vi "ClassPanel.vi"(8 "error in (no error)":errorcluster caption="entrée d'erreur (pas d'erreur)", 11 "CoboltMLD.lvclass":refnum<class "CoboltMLD.lvclass">) -> (0 "error out":errorcluster caption="sortie d'erreur", 3 "CoboltMLD.lvclass Out":refnum<class "CoboltMLD.lvclass">)   [LabVIEW 2019, in "CoboltMLD.lvclass"]
uses:
  CoboltMLD.lvclass
  CoboltModes.ctl
  C:/Programmes Labview/LabscanV1A/DevicesClass/BaseDevice/BaseDevice.lvclass
  <userlib>/TaikoLaser/PDLM_TaggedValueList.ctl
  <userlib>/TaikoLaser/PDLM_TaggedValue.ctl
  <userlib>/TaikoLaser/PDLM_Tag.ctl
  BaseDevice/BaseDevice.lvclass/BaseDevice.ctl
  BaseDevice/ClassQueueMess.ctl
  BaseDevice/Accessor/GetBaseDataPath.vi
  BaseDevice/Accessor/GetClassEvent.vi
panel:
  out "MaxSetpoint":dbl
  in  "Paused":bool
  out "Hours":dbl
  in  "AMod":bool
  out "Fault":string
  in  "DMod":bool
  out "Act Current":dbl caption="Current (mA)" min=0.1 step=0.1 format="%#.3f"
  out "ForceDis":bool caption="Force disconnect"
  out "Error":bool
  out "JournalPath":path
  in  "Con/Disc.":bool
  out "Interlock":bool
  out "Temp":dbl caption="Temp (C)" min=0.1 step=0.1 format="%#.1f"
  out "Act Power":dbl caption="Power (mW)" min=0.1 step=0.1 format="%#.3f"
  in  "Update":bool
  in  "Mode":T1 caption="Laser Mode"
  in  "LaserOn":bool caption="Laser On"
  out "KeyLock":bool
  in  "Setp_Pc":dbl=1.0 caption="Setpoint(%)" min=0.0 max=100.0 step=0.01 format="%#.1f"
  in  "MainProgQ":refnum<queue>
  in  "MainProgQEvent":refnum<user-event>
  in  "Acq":bool
  in  "Stop":bool
  in  "Setp_Un":dbl=200.0 caption="Setpoint(mW)" min=0.0 max=200.0 step=0.01 format="%#.1f"
  out "Init Program":bool
  # "Cobolt Laser"
  # "this MUST labeled with class name"
  # "this MUST be present and labeled \"Stop\" and \"Acq\""
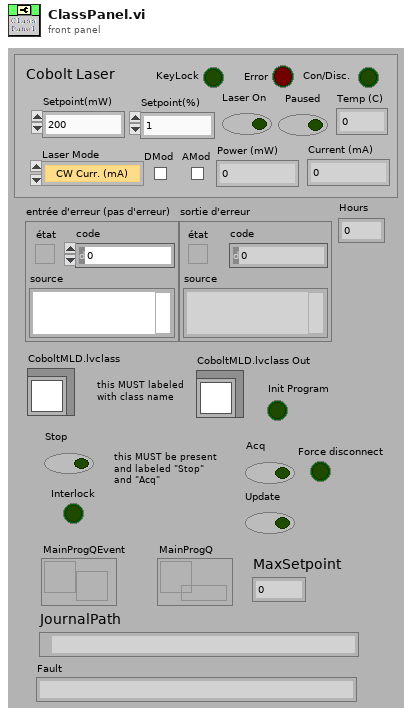
[diagram p1: front panel]
types:
  T1 = typedef "CoboltModes.ctl" = enum16{"CW Curr. (mA)", "CW Pow. (mW)", "Curr. Mod. (mA)", "Pow. Mod. (mW)"}
  T2 = typedef "PDLM_Tag.ctl" = u32
  T3 = typedef "PDLM_TaggedValueList.ctl" = T4[]
  T4 = typedef "PDLM_TaggedValue.ctl" = cluster{"Tag":T2, "Value":u32}
  T5 = typedef "ClassQueueMess.ctl" = u16
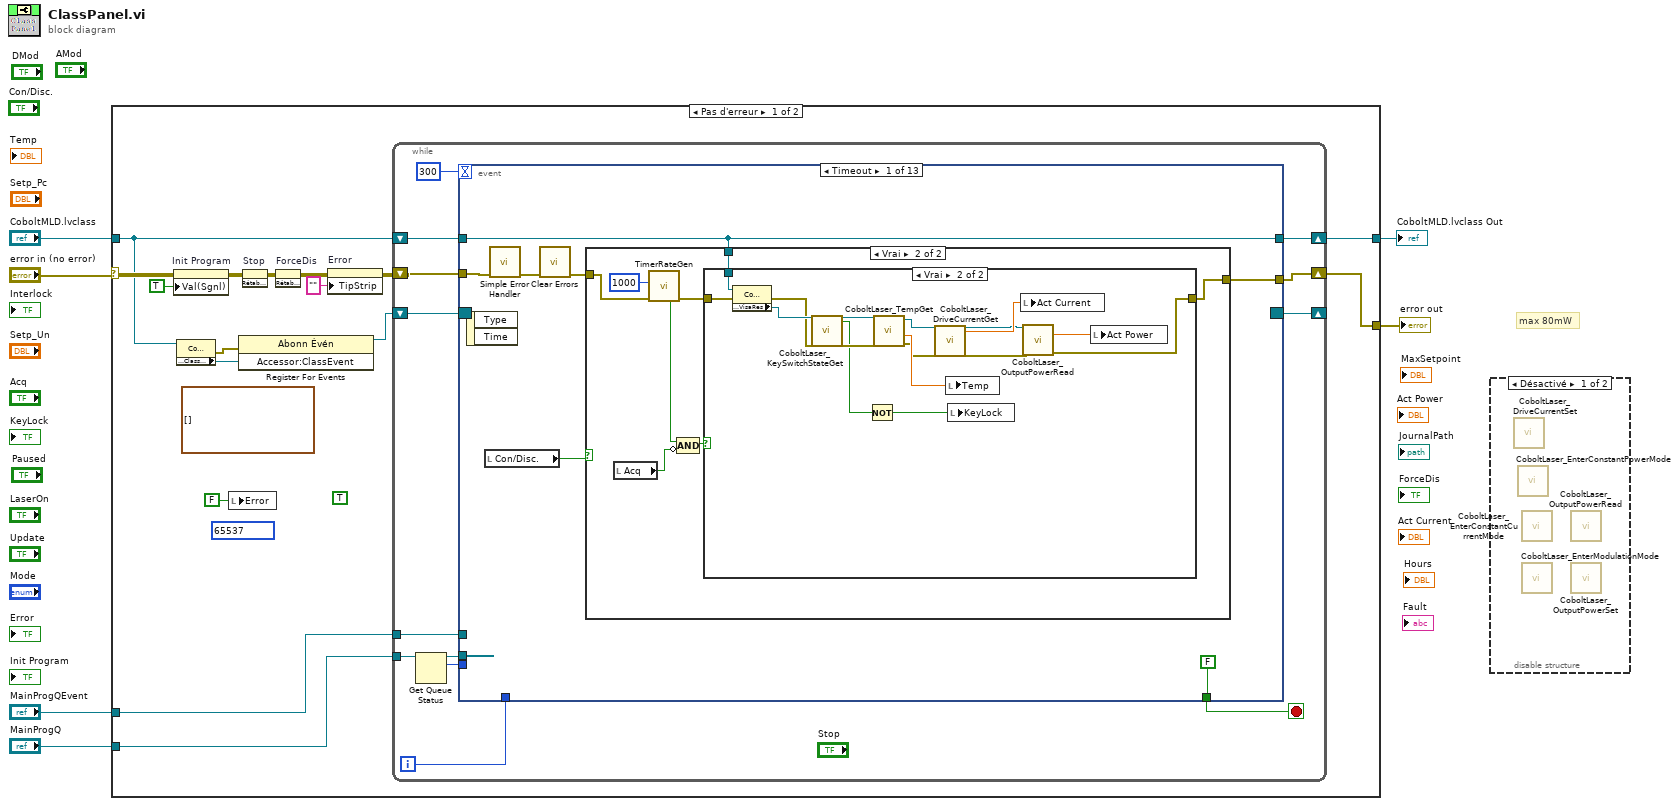
[diagram p0: block diagram]
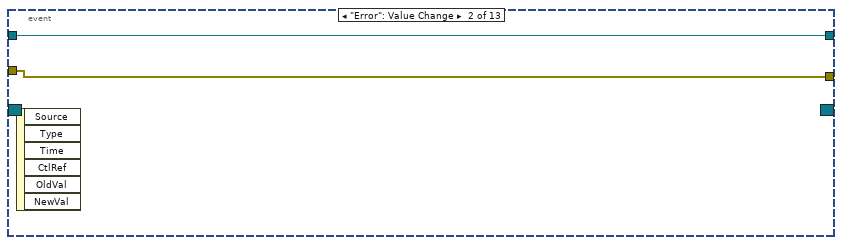
[diagram p5: hidden frame]
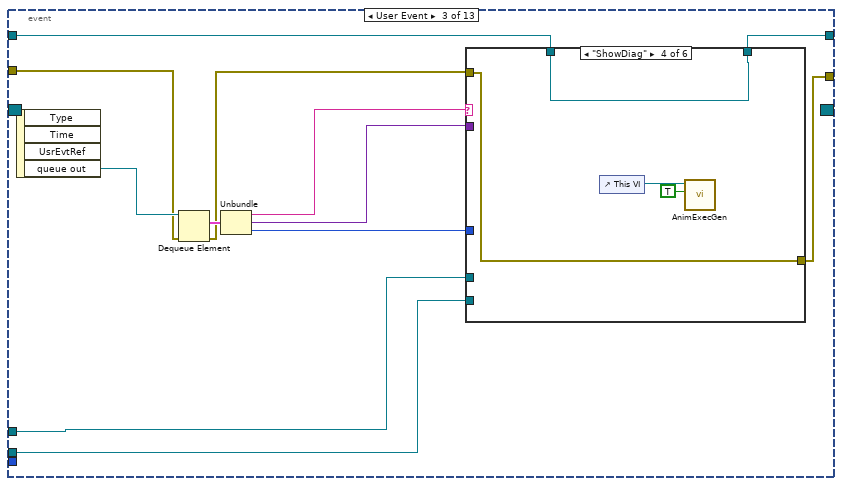
[diagram p6: hidden frame]
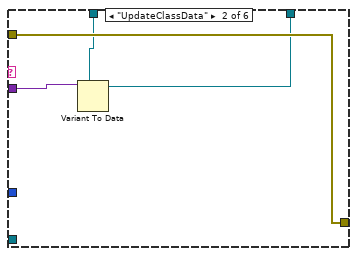
[diagram p8: hidden frame]
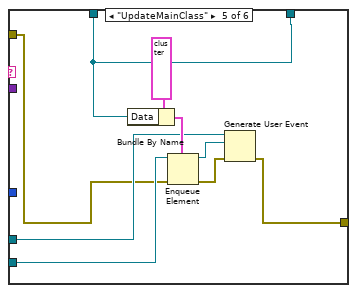
[diagram p10: hidden frame]
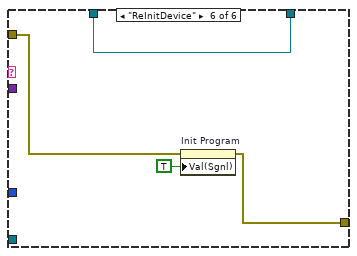
[diagram p11: hidden frame]
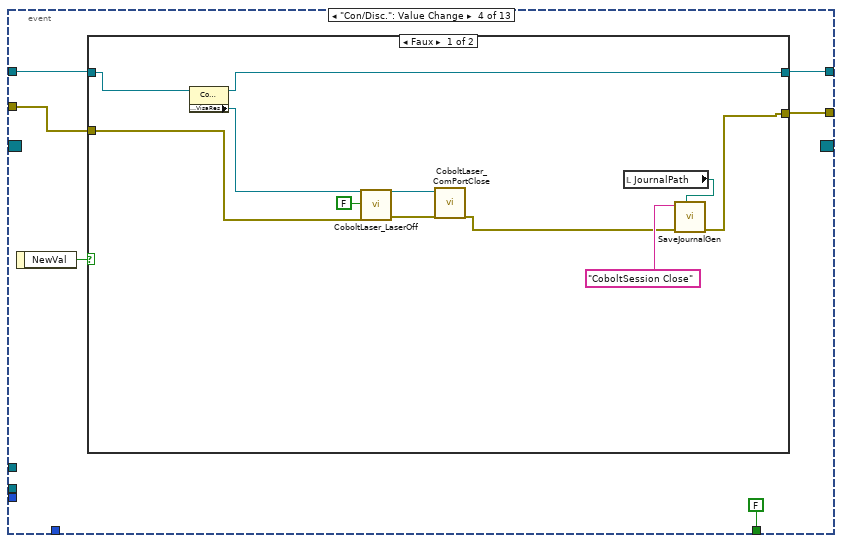
[diagram p12: hidden frame]
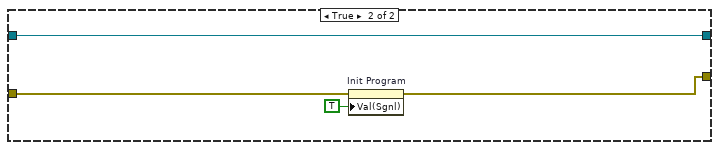
[diagram p13: hidden frame]
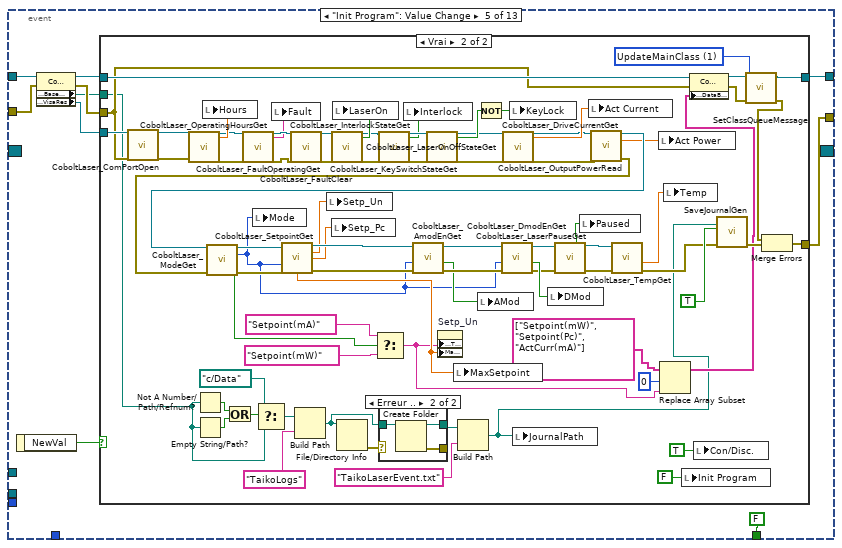
[diagram p14: hidden frame]
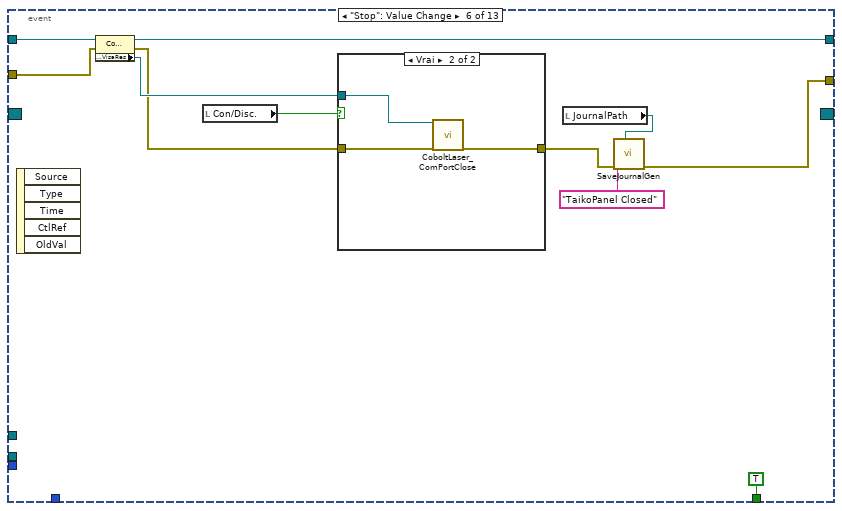
[diagram p17: hidden frame]
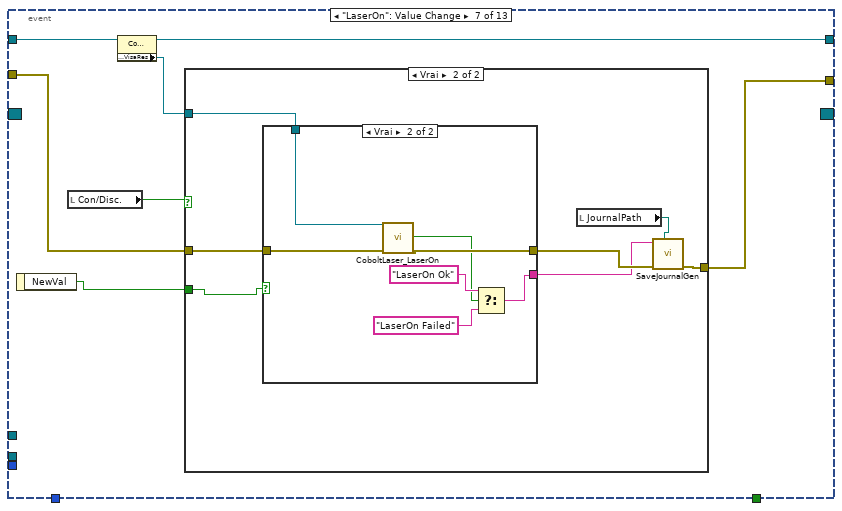
[diagram p19: hidden frame]
diagram:
  # "max 80mW"
  n1 = case shown="Pas d'erreur" "error in (no error)" {
    selector: "error in (no error)" -> [w11 w381]
    tunnel: [w22 w381] -> w5
    tunnel: "CoboltMLD.lvclass" -> [w16 w380]
    tunnel: [w20 w380] -> w3
    tunnel: "MainProgQEvent" -> [w14 _]
    tunnel: "MainProgQ" -> [w13 _]
    frame No Error {
      (unwired) TRUE ("ForceDis")
      (unwired) T2 65537 items=["NONE"=0, "Locked"=16, "SoftLock"=17, "KeyLock"=18, "Class_IV_Lock"=20, "Interlock"=24, "LaserMode"=32, "LDH_PulsePowerTable"=33, "TriggerMode"=48, "TriggerLevelRaw"=64, "TriggerLevelRawLoLimit"=65, "TriggerLevelRawHiLimit"=66, "TriggerLevel"=72, "TriggerLevelLoLimit"=73, "TriggerLevelHiLimit"=74, "FastGate"=80, "FastGateImp"=96, "SlowGate"=112, "TargetTempRaw"=144, "TargetTempRawLoLimit"=145, "TargetTempRawHiLimit"=146, "CurrentTempRaw"=148, "CaseTempRaw"=149, "TargetTemp"=152, "TargetTempLoLimit"=153, "TargetTempHiLimit"=154, "CurrentTemp"=156, "CaseTemp"=157, "TempScale"=159, "Frequency"=168, "FrequencyLoLimit"=169, "FrequencyHiLimit"=170, "PulsePowerRaw"=176, "PulsePowerRawLoLimit"=177, "PulsePowerRawHiLimit"=178, "PulsePowerPermille"=180, "PulseShape"=181, "PulsePower"=184, "PulsePowerLoLimit"=185, "PulsePowerHiLimit"=186, "PulsePowerNanowatt"=188, "PulsePowerVoltage"=190, "PulseEnergy"=191, "CwPowerRaw"=192, "CwPowerRawLoLimit"=193, "CwPowerRawHiLimit"=194, "CwPowerPermille"=196, "CwPower"=200, "CwPowerLoLimit"=201, "CwPowerHiLimit"=202, "CwPowerMicroWatt"=204, "BurstLen"=208, "BurstPeriod"=224, "LDH_Fan"=240, "UI_Exclusive"=256] ("Tag")
      (unwired) T3 [] ("TaggedValueList")
      n2 = property on="Init Program" class="Bool (strict)"(error in=w11, "Val(Sgnl)"=TRUE ("Valeur (Signalisation)")) -> (error out=w19:errorcluster)  [unwired: 1 in, 1 out]
      n3 = property class="CoboltMLD.lvclass"(reference=w16) -> (error out=w18:errorcluster, "Accessor:ClassEvent"=w17:refnum<user-event>)  [unwired: 1 in, 1 out]
      n4 = local write "Error"(FALSE ("Error")) -> ()
      n5 = register-events(error in=w18, w17) -> (reference out=w15:refnum<event-registration>)  [unwired: 1 in, 1 out]
      n6 = invoke on="Stop" class="Bool (strict)" method="RétablirValParDéfaut"(error in=w19) -> (error out=w10:errorcluster)  [unwired: 2 in, 2 out]
      n7 = invoke on="ForceDis" class="Bool (strict)" method="RétablirValParDéfaut"(error in=w10) -> (error out=w9:errorcluster)  [unwired: 2 in, 2 out]
      n8 = property on="Error" class="Bool (strict)"(error in=w9, "TipStrip"="" ("Info-bulle")) -> (error out=w8:errorcluster)  [unwired: 1 in, 1 out]
      n9 = while {
        shift-right: [w33] -> w22
        shift-left: w8 -> [w34]
        shift-right: [w32] -> w20
        shift-left: w16 -> [w26]
        shift-right: [w30] -> _
        shift-left: w15 -> [w31]
        tunnel: w14 -> [w29]
        tunnel: w13 -> [w28]
        i -> [w27]
        stop <- w25 stop-if-true
        n10 = Get Queue Status(queue=w28) -> (queue out=w24:refnum<queue>, # pending remove=w23:i32)  [unwired: 2 in, 6 out]
        n11 = event shown="[0] Timeout" {
          selector: w31 -> [_ _ _ _ _ _ _ _ _ _ _ _ _]
          dyn-events: [_ _ _ _ _ _ _ _ _ _ _ _ _] -> w30
          timeout: 300 -> [_ _ _ _ _ _ _ _ _ _ _ _ _]
          tunnel: w34 -> [w40 w69 w72 w112 w132 w224 w244 w269 w300 w312 w325 w335 w349]
          tunnel: [w37 w69 w76 w109 w137 w229 w242 w271 w298 w310 w323 w334 w346] -> w33
          tunnel: w26 -> [w36 w70 w82 w110 w135 w232 w243 w272 w299 w311 w324 w337 w350]
          tunnel: [FALSE _ _ FALSE FALSE TRUE _ _ _ _ _ _ _] -> w25
          tunnel: [w36 w70 w75 w108 w134 w226 w241 w270 w299 w311 w324 w337 w343] -> w32
          tunnel: w29 -> [_ _ w74 _ _ _ _ _ _ _ _ _ _]
          tunnel: w24 -> [_ _ w73 _ _ _ _ _ _ _ _ _ _]
          tunnel: w27 -> [_ _ _ _ _ _ _ _ _ _ _ _ _]
          tunnel: w23 -> [_ _ _ _ _ _ _ _ _ _ _ _ _]
          event Timeout {
            n12 = event-data() -> ()  [unwired: 1 in, 2 out]
            n13 = local read "Con/Disc."() -> (w38:bool)
            n14 = call <vilib>:"Simple Error Handler.vi"("error in (no error)"=w40) -> ("error out"=w41:errorcluster)  [unwired: 4 in, 4 out]
            n15 = call <vilib>:"Clear Errors.vi"("error in (no error)"=w41) -> ("error out"=w39:errorcluster)  [unwired: 5 in, 1 out]
            n16 = case shown="Vrai" w38 {
              tunnel: w39 -> [w43 w51]
              tunnel: [w43 w47] -> w37
              tunnel: w36 -> [_ w46]
              frame False {
              }
              frame True {
                n17 = local read "Acq"() -> (w44:bool)
                n18 = call <userlib>:"TimerRateGen.vi"("error in (no error)"=w51, "Refresh(ms)"=u32 1000) -> ("error out"=w49:errorcluster, "updated?"=w48:bool)  [unwired: 7 in, 1 out]
                n19 = Compound Arithmetic op=AND ("Opérateur arithmétique")(w48, invert w44) -> (w45:bool)
                n20 = case shown="Vrai" w45 {
                  tunnel: w49 -> [w52 w68]
                  tunnel: [w52 w53] -> w47
                  tunnel: w46 -> [_ w64]
                  frame False {
                  }
                  frame True {
                    n21 = property class="CoboltMLD.lvclass"(reference=w64, error in=w68) -> (error out=w65:errorcluster, "Accessor:VisaRes"=w67:refnum<visa-resource-name>)  [unwired: 1 out]
                    n22 = call <userlib>:"CoboltLaser_KeySwitchStateGet.vi"("ComPort"=w67, "error in (no error)"=w65) -> ("ComPortOut"=w66:refnum<visa-resource-name>, "Enable"=w61:bool, "error out"=w63:errorcluster)  [unwired: 23 in]
                    n23 = Not(x=w61) -> (.not. x?=w60:bool)
                    n24 = call <userlib>:"CoboltLaser_TempGet.vi"("ErrorIn"=w63, "ComPort"=w66) -> ("ErrorOut"=w54:errorcluster, "Température"=w62:dbl, "ComPortOut"=w55:refnum<visa-resource-name>)  [unwired: 5 in, 2 out]
                    n25 = call <userlib>:"CoboltLaser_DriveCurrentGet.vi"("ComPort"=w55, "ErrorIn"=w54) -> ("ComPortOut"=w57:refnum<visa-resource-name>, "LaserCurrent"=w59:dbl, "ErrorOut"=w58:errorcluster)  [unwired: 23 in]
                    n26 = local write "Temp"(w62) -> ()
                    n27 = local write "KeyLock"(w60) -> ()
                    n28 = local write "Act Current"(w59) -> ()
                    n29 = call <userlib>:"CoboltLaser_OutputPowerRead.vi"("ComPort"=w57, "ErrorIn"=w58) -> ("OutputPower"=w56:dbl, "ErrorOut"=w53:errorcluster)  [unwired: 11 in, 1 out]
                    n30 = local write "Act Power"(w56) -> ()
                  }
                }
              }
            }
          }
          event "Error": Value Change {
            n31 = event-data() -> ()  [unwired: 1 in, 6 out]
          }
          event User Event {
            n32 = event-data() -> ("queue out"=w80:refnum<queue>)  [unwired: 1 in, 3 out]
            n33 = Dequeue Element(queue=w80, error in (no error)=w72) -> (element=w81:cluster{"Message":string, "Data":variant, i32}, error out=w71:errorcluster)  [unwired: 1 in, 2 out]
            n34 = Unbundle(w81) -> ("Message"=w79:string, "Data"=w78:variant, w77:i32)
            n35 = case shown="\"ShowDiag\"" w79 {
              tunnel: w71 -> [w84 w88 w89 w93 w96 w106]
              tunnel: w78 -> [_ w87 _ _ _ _]
              tunnel: w82 -> [w83 w86 w90 w94 w99 w107]
              tunnel: [w83 w85 w90 w94 w99 w107] -> w75
              tunnel: [w84 w88 w89 w93 w95 w105] -> w76
              tunnel: w77 -> [_ _ _ _ _ _]
              tunnel: w74 -> [_ _ _ _ w98 _]
              tunnel: w73 -> [_ _ _ _ w97 _]
              frame Default {
              }
              frame "UpdateClassData" {
                n36 = Variant To Data(type=w86, Variant=w87) -> (data=w85:refnum<class "CoboltMLD.lvclass">)  [unwired: 1 in, 1 out]
              }
              frame "MeasDone" {
              }
              frame "ShowDiag" {
                n37 = control-ref of="This VI"() -> (w92:refnum<vi>)
                n38 = call <userlib>:"AnimExecGen.vi"("Animer l'exécution ?"=TRUE, "ViRef"=w92) -> ()  [unwired: 9 in, 1 out]
              }
              frame "UpdateMainClass" {
                n39 = Bundle By Name(cluster=cluster{"Message":string, "Data":variant, i32} {"Message"="", "Data"=variant, 0} ("élément"), "Data"=w99) -> (w100:cluster{"Message":string, "Data":variant, i32})
                n40 = Enqueue Element(queue=w97, element=w100, error in (no error)=w96) -> (queue out=w103:refnum<queue>, error out=w102:errorcluster)  [unwired: 1 in, 1 out]
                n41 = Generate User Event(user event=w98, event data cluster=w103, error in=w102) -> (error out=w95:errorcluster)  [unwired: 1 in, 1 out]
              }
              frame "ReInitDevice" {
                n42 = property on="Init Program" class="Bool (strict)"(error in=w106, "Val(Sgnl)"=TRUE ("Valeur (Signalisation)")) -> (error out=w105:errorcluster)  [unwired: 1 in, 1 out]
              }
            }
          }
          event "Con/Disc.": Value Change {
            n43 = event-data() -> ("NewVal"=w111:bool)  [unwired: 1 in]
            n44 = case shown="Faux" w111 {
              tunnel: w112 -> [w115 w127]
              tunnel: w110 -> [w120 w128]
              tunnel: [w119 w128] -> w108
              tunnel: [w122 w125] -> w109
              frame False {
                n45 = property class="CoboltMLD.lvclass"(reference=w120) -> (reference out=w119:refnum<class "CoboltMLD.lvclass">, "Accessor:VisaRes"=w118:refnum<visa-resource-name>)  [unwired: 1 in, 1 out]
                n46 = call <userlib>:"CoboltLaser_LaserOff.vi"("ComPort"=w118, "GenerateError"=FALSE, "error in (no error)"=w115) -> ("ComPortOut"=w117:refnum<visa-resource-name>, "error out"=w116:errorcluster)  [unwired: 21 in, 2 out]
                n47 = call <userlib>:"CoboltLaser_ComPortClose.vi"("ComPort"=w117, "error in (no error)"=w116) -> ("error out"=w121:errorcluster)  [unwired: 17 in]
                n48 = local read "JournalPath"() -> (w124:path)
                n49 = call <userlib>:"SaveJournalGen.vi"("CheminSauv"=w124, "error in"=w121, "Journal Text"="CoboltSession Close") -> ("error out"=w122:errorcluster)  [unwired: 7 in, 1 out]
              }
              frame True {
                n50 = property on="Init Program" class="Bool (strict)"(error in=w127, "Val(Sgnl)"=TRUE ("Valeur (Signalisation)")) -> (error out=w125:errorcluster)  [unwired: 1 in, 1 out]
              }
            }
          }
          event "Init Program": Value Change {
            n51 = event-data() -> ("NewVal"=w138:bool)  [unwired: 1 in]
            n52 = property class="CoboltMLD.lvclass"(reference=w135, error in=w132) -> (reference out=w133:refnum<class "CoboltMLD.lvclass">, error out=w131:errorcluster, "Accessor:BaseDataPath"=w129:path, "Accessor:VisaRes"=w130:refnum<visa-resource-name>)
            n53 = case shown="Vrai" w138 {
              tunnel: w131 -> [w140 w157]
              tunnel: [w140 w160] -> w137
              tunnel: w133 -> [w139 w165]
              tunnel: [w139 w163] -> w134
              tunnel: w130 -> [_ w216]
              tunnel: w129 -> [_ w142]
              frame False {
              }
              frame True {
                w162 = T5 1 items=["UpdateClassData", "UpdateMainClass", "UpdateDataBind", "ReInitDevice", "Custom", "ClosePan"] ("Menu déroulant")
                n54 = call <userlib>:"CoboltLaser_ComPortOpen.vi"("ComPort"=w216, "error in (no error)"=w157) -> ("ComPort Out"=w214:refnum<visa-resource-name>, "error out"=w215:errorcluster)  [unwired: 16 in]
                n55 = call <userlib>:"CoboltLaser_OperatingHoursGet.vi"("ComPort"=w214, "error in (no error)"=w215) -> ("ComPortOut"=w203:refnum<visa-resource-name>, "OperatingHours"=w205:dbl, "error out"=w204:errorcluster)  [unwired: 23 in]
                n56 = Not A Number/Path/Refnum?(number/path/refnum=w142) -> (NaN/Path/Refnum?=w147:bool)
                n57 = Empty String/Path?(string/path=w142) -> (empty?=w146:bool)
                n58 = local write "Hours"(w205) -> ()
                n59 = Or(x=w147, y=w146) -> (x .or. y?=w145:bool)
                n60 = call <userlib>:"CoboltLaser_FaultOperatingGet.vi"("ComPort"=w203, "error in (no error)"=w204) -> ("ComPortOut"=w206:refnum<visa-resource-name>, "Fault"=w197:string, "error out"=w207:errorcluster)  [unwired: 23 in]
                n61 = Select(t=path "c:/Data" ("cas vrai"), s=w145, f=w142) -> (s? t:f=w143:path)
                n62 = local write "Fault"(w197) -> ()
                n63 = call <userlib>:"CoboltLaser_FaultClear.vi"("ComPort"=w206, "error in (no error)"=w207) -> ("ComPortOut"=w202:refnum<visa-resource-name>, "error out"=w201:errorcluster)  [unwired: 24 in]
                n64 = Build Path(base path=w143, name or relative path="TaikoLogs" ("nom ou chemin relatif")) -> (appended path=w150:path)
                n65 = call <userlib>:"CoboltLaser_LaserOnOffStateGet.vi"("ComPort"=w202, "error in (no error)"=w201) -> ("ComPortOut"=w199:refnum<visa-resource-name>, "On"=w200:bool, "error out"=w198:errorcluster)  [unwired: 21 in, 2 out]
                n66 = local write "LaserOn"(w200) -> ()
                n67 = File/Directory Info(path=w150) -> (error out=w151:errorcluster)  [unwired: 1 in, 6 out]
                n68 = call <userlib>:"CoboltLaser_InterlockStateGet.vi"("ComPort"=w199, "error in (no error)"=w198) -> ("ComPortOut"=w213:refnum<visa-resource-name>, "InterlockOpen"=w212:bool, "error out"=w211:errorcluster)  [unwired: 23 in]
                n69 = case shown="Erreur .." w151 {
                  selector: w151 -> [w219 _]
                  tunnel: w150 -> [w218 w222]
                  tunnel: [w219 w221] -> _
                  tunnel: [w218 w220] -> w149
                  frame No Error {
                  }
                  frame Error {
                    n70 = Create Folder(path (use dialog)=w222) -> (created path=w220:path, error out=w221:errorcluster)  [unwired: 2 in, 1 out]
                  }
                }
                n71 = local write "Interlock"(w212) -> ()
                n72 = call <userlib>:"CoboltLaser_KeySwitchStateGet.vi"("ComPort"=w213, "error in (no error)"=w211) -> ("ComPortOut"=w195:refnum<visa-resource-name>, "Enable"=w210:bool, "error out"=w196:errorcluster)  [unwired: 23 in]
                n73 = Build Path(base path=w149, name or relative path="TaikoLaserEvent.txt" ("nom ou chemin relatif")) -> (appended path=w141:path)
                n74 = Not(x=w210) -> (.not. x?=w209:bool)
                n75 = call <userlib>:"CoboltLaser_DriveCurrentGet.vi"("ComPort"=w195, "ErrorIn"=w196) -> ("ComPortOut"=w178:refnum<visa-resource-name>, "LaserCurrent"=w194:dbl, "ErrorOut"=w179:errorcluster)  [unwired: 23 in]
                n76 = local write "KeyLock"(w209) -> ()
                n77 = local write "JournalPath"(w141) -> ()
                n78 = local write "Act Current"(w194) -> ()
                n79 = call <userlib>:"CoboltLaser_OutputPowerRead.vi"("ComPort"=w178, "ErrorIn"=w179) -> ("ComPortOut"=w177:refnum<visa-resource-name>, "OutputPower"=w175:dbl, "ErrorOut"=w176:errorcluster)  [unwired: 11 in]
                n80 = call <userlib>:"CoboltLaser_ModeGet.vi"("ComPort"=w177, "ErrorIn"=w176) -> ("ComPortOut"=w192:refnum<visa-resource-name>, "Mode"=w166:T1, "Units(mA:1)"=w184:bool, "ErrorOut"=w191:errorcluster)  [unwired: 9 in, 1 out]
                n81 = local write "Mode"(w166) -> ()
                n82 = call <userlib>:"CoboltLaser_SetpointGet.vi"("ComPort"=w192, "Mode"=w166, "ErrorIn"=w191) -> ("ComPortOut"=w189:refnum<visa-resource-name>, "Setpoint_Un"=w181:dbl, "Setpoint_Pc"=w180:dbl, "MaxSetpoint"=w171:dbl, "ErrorOut"=w190:errorcluster)  [unwired: 5 in, 3 out]
                n83 = local write "Setp_Un"(w181) -> ()
                n84 = local write "Setp_Pc"(w180) -> ()
                n85 = Select(t="Setpoint(mA)" ("Sous-titre.Texte"), s=w184, f="Setpoint(mW)" ("Sous-titre.Texte")) -> (s? t:f=w155:string)
                n86 = call <userlib>:"CoboltLaser_AmodEnGet.vi"("ErrorIn"=w190, "Mode"=w166, "ComPort"=w189) -> ("ErrorOut"=w188:errorcluster, "Enabled"=w185:bool, "ComPortOut"=w187:refnum<visa-resource-name>)  [unwired: 4 in, 2 out]
                n87 = property on="Setp_Un" class="NumNb (strict)"("Caption.Text"=w155, "Maximum"=w171) -> ()  [unwired: 2 in, 2 out]
                n88 = local write "MaxSetpoint"(w171) -> ()
                n89 = local write "AMod"(w185) -> ()
                n90 = call <userlib>:"CoboltLaser_DmodEnGet.vi"("ErrorIn"=w188, "Mode"=w166, "ComPort"=w187) -> ("ErrorOut"=w174:errorcluster, "Enabled"=w186:bool, "ComPortOut"=w173:refnum<visa-resource-name>)  [unwired: 4 in, 2 out]
                n91 = local write "DMod"(w186) -> ()
                n92 = call <userlib>:"CoboltLaser_LaserPauseGet.vi"("ComPort"=w173, "error in (no error)"=w174) -> ("Paused"=w172:bool, "ComPortOut"=w169:refnum<visa-resource-name>, "error out"=w170:errorcluster)  [unwired: 9 in, 2 out]
                n93 = local write "Paused"(w172) -> ()
                n94 = call <userlib>:"CoboltLaser_TempGet.vi"("ErrorIn"=w170, "ComPort"=w169) -> ("ErrorOut"=w168:errorcluster, "Température"=w167:dbl)  [unwired: 5 in, 3 out]
                n95 = local write "Act Power"(w175) -> ()
                n96 = Replace Array Subset(array=string[] ["Setpoint(mW)", "Setpoint(Pc)", "ActCurr(mA)"], new element=w155, index=0 ("indice")) -> (w154:string[])
                n97 = local write "Temp"(w167) -> ()
                n98 = local write "Init Program"(FALSE ("Init Program")) -> ()
                n99 = property class="CoboltMLD.lvclass"(reference=w165, error in=w157, "Accessor:DataBindCtrl"=w154) -> (reference out=w164:refnum<class "CoboltMLD.lvclass">, error out=w161:errorcluster)
                n100 = local write "Con/Disc."(TRUE ("Con/Disc.")) -> ()
                n101 = call <userlib>:"SaveJournalGen.vi"("CheminSauv"=w141, "error in"=w168, "Include Date_Time"=TRUE) -> ("error out"=w159:errorcluster)  [unwired: 7 in, 1 out]
                n102 = call-dynamic "SetClassQueueMessage.vi"("ErrorIn(No Error)"=w161, "Menu déroulant"=w162, "DefaultDev.lvclass"=w164) -> ("sortie d'erreur"=w158:errorcluster, "DefaultDev.lvclass Out"=w163:refnum<class "CoboltMLD.lvclass">)  [unwired: 7 in]
                n103 = Merge Errors(w158, w159) -> (w160:errorcluster)
              }
            }
          }
          event "Stop": Value Change {
            n104 = event-data() -> ()  [unwired: 1 in, 5 out]
            n105 = property class="CoboltMLD.lvclass"(reference=w232, error in=w224) -> (reference out=w226:refnum<class "CoboltMLD.lvclass">, error out=w223:errorcluster, "Accessor:VisaRes"=w225:refnum<visa-resource-name>)
            n106 = local read "Con/Disc."() -> (w227:bool)
            n107 = case shown="Vrai" w227 {
              tunnel: w223 -> [w234 w237]
              tunnel: [w234 w236] -> w230
              tunnel: w225 -> [_ w235]
              frame False {
              }
              frame True {
                n108 = call <userlib>:"CoboltLaser_ComPortClose.vi"("ComPort"=w235, "error in (no error)"=w237) -> ("error out"=w236:errorcluster)  [unwired: 17 in]
              }
            }
            n109 = local read "JournalPath"() -> (w231:path)
            n110 = call <userlib>:"SaveJournalGen.vi"("CheminSauv"=w231, "error in"=w230, "Journal Text"="TaikoPanel Closed") -> ("error out"=w229:errorcluster)  [unwired: 7 in, 1 out]
          }
          event "LaserOn": Value Change {
            n111 = event-data() -> ("NewVal"=w238:bool)  [unwired: 1 in]
            n112 = local read "Con/Disc."() -> (w240:bool)
            n113 = property class="CoboltMLD.lvclass"(reference=w243) -> (reference out=w241:refnum<class "CoboltMLD.lvclass">, "Accessor:VisaRes"=w239:refnum<visa-resource-name>)  [unwired: 1 in, 1 out]
            n114 = case shown="Vrai" w240 {
              tunnel: w244 -> [w245 w249]
              tunnel: [w245 w252] -> w242
              tunnel: w239 -> [_ w247]
              tunnel: w238 -> [_ w250]
              frame False {
              }
              frame True {
                n115 = case shown="Vrai" w250 {
                  tunnel: w249 -> [w259 w266]
                  tunnel: [w258 w265] -> w248
                  tunnel: [w253 w261] -> w246
                  tunnel: w247 -> [w257 w260]
                  frame False {
                    n116 = call <userlib>:"CoboltLaser_LaserOff.vi"("ComPort"=w257, "error in (no error)"=w259) -> ("ResponseOK"=w256:bool, "error out"=w258:errorcluster)  [unwired: 22 in, 2 out]
                    n117 = Select(t="LaserOff Ok" ("chaîne de format"), s=w256, f="LaserOff Failed" ("chaîne de format")) -> (s? t:f=w253:string)
                  }
                  frame True {
                    n118 = call <userlib>:"CoboltLaser_LaserOn.vi"("ComPort"=w260, "error in (no error)"=w266) -> ("ResponseOK"=w263:bool, "error out"=w265:errorcluster)  [unwired: 22 in, 2 out]
                    n119 = Select(t="LaserOn Ok" ("chaîne de format"), s=w263, f="LaserOn Failed" ("chaîne de format")) -> (s? t:f=w261:string)
                  }
                }
                n120 = local read "JournalPath"() -> (w251:path)
                n121 = call <userlib>:"SaveJournalGen.vi"("CheminSauv"=w251, "error in"=w248, "Journal Text"=w246) -> ("error out"=w252:errorcluster)  [unwired: 7 in, 1 out]
              }
            }
          }
          event "Setp_Un": Value Change {
            n122 = event-data() -> ("NewVal"=w268:dbl)  [unwired: 1 in]
            n123 = local read "Con/Disc."() -> (w267:bool)
            n124 = case shown="Vrai" w267 {
              tunnel: w272 -> [w274 w284]
              tunnel: [w273 w283] -> w271
              tunnel: [w274 w282] -> w270
              tunnel: w269 -> [w273 w281]
              tunnel: w268 -> [_ w277]
              frame False {
              }
              frame True {
                n125 = property class="CoboltMLD.lvclass"(reference=w284, error in=w281) -> (reference out=w282:refnum<class "CoboltMLD.lvclass">, error out=w279:errorcluster, "Accessor:VisaRes"=w280:refnum<visa-resource-name>)
                n126 = local read "Mode"() -> (w275:T1)
                n127 = call <userlib>:"CoboltLaser_SetpointSet.vi"("ComPort"=w280, "Setpoint_Un"=w277, "Mode"=w275, "ErrorIn"=w279) -> ("Setpoint_Pc"=w276:dbl, "ErrorOut"=w278:errorcluster)  [unwired: 5 in, 5 out]
                n128 = case shown="Pas d'erreur" w278 {
                  selector: w278 -> [w290 w295]
                  tunnel: [w291 w295] -> w283
                  tunnel: w277 -> [w289 _]
                  tunnel: w276 -> [w288 _]
                  tunnel: w275 -> [w286 _]
                  frame No Error {
                    n129 = Index Array(array=string[] ["SetCWCurrent %.2f mA; %.2f Pc", "SetCWPower %.2f mW; %.2f Pc", "SetModCurrent %.2f mA; %.2f Pc", "SetModPower %.2f mW; %.2f Pc"], index=w286) -> (element=w285:string)
                    n130 = Format Into String(format string=w285, error in=w290, w289, w288) -> (resulting string=w294:string, error out=w292:errorcluster)  [unwired: 1 in]
                    n131 = local read "JournalPath"() -> (w293:path)
                    n132 = call <userlib>:"SaveJournalGen.vi"("CheminSauv"=w293, "error in"=w292, "Journal Text"=w294) -> ("error out"=w291:errorcluster)  [unwired: 7 in, 1 out]
                  }
                  frame Error {
                  }
                }
              }
            }
          }
          event "Paused": Value Change {
            n133 = event-data() -> ("NewVal"=w296:bool)  [unwired: 1 in]
            n134 = local read "Con/Disc."() -> (w297:bool)
            n135 = case shown="Vrai" w297 {
              tunnel: w299 -> [_ w307]
              tunnel: w300 -> [w301 w306]
              tunnel: [w301 w302] -> w298
              tunnel: w296 -> [_ w304]
              frame False {
              }
              frame True {
                n136 = property class="CoboltMLD.lvclass"(reference=w307, error in=w306) -> (error out=w303:errorcluster, "Accessor:VisaRes"=w305:refnum<visa-resource-name>)  [unwired: 1 out]
                n137 = call <userlib>:"CoboltLaser_LaserPauseSet.vi"("ComPort"=w305, "Paused"=w304, "error in (no error)"=w303) -> ("error out"=w302:errorcluster)  [unwired: 10 in, 2 out]
              }
            }
          }
          event "DMod": Value Change {
            n138 = event-data() -> ("NewVal"=w308:bool)  [unwired: 1 in]
            n139 = local read "Con/Disc."() -> (w309:bool)
            n140 = case shown="Vrai" w309 {
              tunnel: w311 -> [_ w320]
              tunnel: w312 -> [w313 w319]
              tunnel: [w313 w316] -> w310
              tunnel: w308 -> [_ w315]
              frame False {
              }
              frame True {
                n141 = property class="CoboltMLD.lvclass"(reference=w320, error in=w319) -> (error out=w317:errorcluster, "Accessor:VisaRes"=w318:refnum<visa-resource-name>)  [unwired: 1 out]
                n142 = local read "Mode"() -> (w314:T1)
                n143 = call <userlib>:"CoboltLaser_DmodEnSet.vi"("Mode"=w314, "ErrorIn"=w317, "Enabled"=w315, "ComPort"=w318) -> ("ErrorOut"=w316:errorcluster)  [unwired: 3 in, 4 out]
              }
            }
          }
          event "AMod": Value Change {
            n144 = event-data() -> ("NewVal"=w321:bool)  [unwired: 1 in]
            n145 = local read "Con/Disc."() -> (w322:bool)
            n146 = case shown="Vrai" w322 {
              tunnel: w324 -> [_ w333]
              tunnel: w325 -> [w326 w332]
              tunnel: [w326 w329] -> w323
              tunnel: w321 -> [_ w328]
              frame False {
              }
              frame True {
                n147 = property class="CoboltMLD.lvclass"(reference=w333, error in=w332) -> (error out=w330:errorcluster, "Accessor:VisaRes"=w331:refnum<visa-resource-name>)  [unwired: 1 out]
                n148 = local read "Mode"() -> (w327:T1)
                n149 = call <userlib>:"CoboltLaser_AmodEnSet.vi"("Mode"=w327, "ErrorIn"=w330, "Enabled"=w328, "ComPort"=w331) -> ("ErrorOut"=w329:errorcluster)  [unwired: 3 in, 4 out]
              }
            }
          }
          event "Setp_Pc": Value Change {
            n150 = event-data() -> ("NewVal"=w341:dbl)  [unwired: 1 in]
            n151 = local read "MaxSetpoint"() -> (w338:dbl)
            n152 = Divide(x=w341, y=100.0) -> (x/y=w340:dbl)
            n153 = Multiply(x=w340, y=w338) -> (x*y=w336:dbl)
            n154 = property on="Setp_Un" class="NumNb (strict)"(error in=w335, "Val(Sgnl)"=w336) -> (error out=w334:errorcluster)  [unwired: 1 in, 1 out]
          }
          event Value Change {
            n155 = event-data() -> ("NewVal"=w348:T1)  [unwired: 1 in]
            n156 = property class="CoboltMLD.lvclass"(reference=w350, error in=w349) -> (reference out=w342:refnum<class "CoboltMLD.lvclass">, error out=w345:errorcluster, "Accessor:VisaRes"=w344:refnum<visa-resource-name>)
            n157 = local read "Con/Disc."() -> (w347:bool)
            n158 = case shown="Vrai" w347 {
              tunnel: w348 -> [_ w363]
              tunnel: [w352 w354] -> w346
              tunnel: w345 -> [w352 w372]
              tunnel: w344 -> [_ w373]
              tunnel: [w351 w356] -> w343
              tunnel: w342 -> [w351 w362]
              frame False {
              }
              frame True {
                w353 = T5 1 items=["UpdateClassData", "UpdateMainClass", "UpdateDataBind", "ReInitDevice", "Custom", "ClosePan"] ("Menu déroulant")
                n159 = call <userlib>:"CoboltLaser_ModeSet.vi"("ComPort"=w373, "Mode"=w363, "ErrorIn"=w372) -> ("ComPortOut"=w371:refnum<visa-resource-name>, "ErrorOut"=w370:errorcluster)  [unwired: 9 in, 2 out]
                n160 = call <userlib>:"CoboltLaser_DmodEnGet.vi"("ErrorIn"=w370, "Mode"=w363, "ComPort"=w371) -> ("ErrorOut"=w369:errorcluster, "Enabled"=w367:bool, "ComPortOut"=w368:refnum<visa-resource-name>)  [unwired: 4 in, 2 out]
                n161 = local write "DMod"(w367) -> ()
                n162 = call <userlib>:"CoboltLaser_AmodEnGet.vi"("ErrorIn"=w369, "Mode"=w363, "ComPort"=w368) -> ("ErrorOut"=w365:errorcluster, "Enabled"=w366:bool, "ComPortOut"=w364:refnum<visa-resource-name>)  [unwired: 4 in, 2 out]
                n163 = local write "AMod"(w366) -> ()
                n164 = call <userlib>:"CoboltLaser_SetpointGet.vi"("ComPort"=w364, "Mode"=w363, "ErrorIn"=w365) -> ("Setpoint_Un"=w374:dbl, "Setpoint_Pc"=w375:dbl, "Units(mW:F)"=w376:bool, "MaxSetpoint"=w377:dbl, "ErrorOut"=w355:errorcluster)  [unwired: 5 in, 3 out]
                n165 = local write "Setp_Pc"(w375) -> ()
                n166 = local write "Setp_Un"(w374) -> ()
                n167 = Select(t="Setpoint(mA)" ("Sous-titre.Texte"), s=w376, f="Setpoint(mW)" ("Sous-titre.Texte")) -> (s? t:f=w359:string)
                n168 = Replace Array Subset(array=string[] ["Setpoint(mW)", "Setpoint(Pc)", "ActCurr(mA)"], new element=w359, index=0 ("indice")) -> (w358:string[])
                n169 = property on="Setp_Un" class="NumNb (strict)"("Caption.Text"=w359, "Maximum"=w377) -> ()  [unwired: 2 in, 2 out]
                n170 = local write "MaxSetpoint"(w377) -> ()
                n171 = property class="CoboltMLD.lvclass"(reference=w362, "Accessor:DataNames"=w358) -> (reference out=w357:refnum<class "CoboltMLD.lvclass">)  [unwired: 1 in, 1 out]
                n172 = call-dynamic "SetClassQueueMessage.vi"("ErrorIn(No Error)"=w355, "Menu déroulant"=w353, "DefaultDev.lvclass"=w357) -> ("sortie d'erreur"=w354:errorcluster, "DefaultDev.lvclass Out"=w356:refnum<class "CoboltMLD.lvclass">)  [unwired: 7 in]
              }
            }
          }
        }
      }
    }
    frame Error {
    }
  }
  "error out" <- w5
  "CoboltMLD.lvclass Out" <- w3
  n173 = disable-structure shown="Désactivé" {
    frame Disabled {
      n174 = call <userlib>:"CoboltLaser_DriveCurrentSet.vi"() -> ()  [unwired: 26 in, 2 out]
      n175 = call <userlib>:"CoboltLaser_EnterConstantPowerMode.vi"() -> ()  [unwired: 26 in, 2 out]
      n176 = call <userlib>:"CoboltLaser_EnterConstantCurrentMode.vi"() -> ()  [unwired: 26 in, 2 out]
      n177 = call <userlib>:"CoboltLaser_EnterModulationMode.vi"() -> ()  [unwired: 26 in, 2 out]
      n178 = call <userlib>:"CoboltLaser_OutputPowerRead.vi"() -> ()  [unwired: 25 in, 3 out]
      n179 = call <userlib>:"CoboltLaser_OutputPowerSet.vi"() -> ()  [unwired: 26 in, 2 out]
    }
    frame Enabled {
    }
  }
